vi "Write ADU Packet.vi"(8 "error in":errorcluster, 9 "modbus data unit":refnum<class "Modbus Data Unit.lvclass">, 10 "protocol layer":refnum<class "Network Protocol.lvclass">, 11 "transmission data unit in":refnum<class "Transmission Data Unit.lvclass">) -> (0 "error out":errorcluster, 2 "protocol layer out":refnum<class "Network Protocol.lvclass">, 3 "transmission data unit out":refnum<class "Transmission Data Unit.lvclass">)   [LabVIEW 2012, in "Transmission Data Unit.lvclass"]
doc: "This method accepts a modbus modbus data unit as input and writes the data of the PDU onto the selected network."
uses:
  Transmission Data Unit.lvclass
  Modbus Data Unit/Modbus Data Unit.lvclass
  Network Protocol/Network Protocol.lvclass
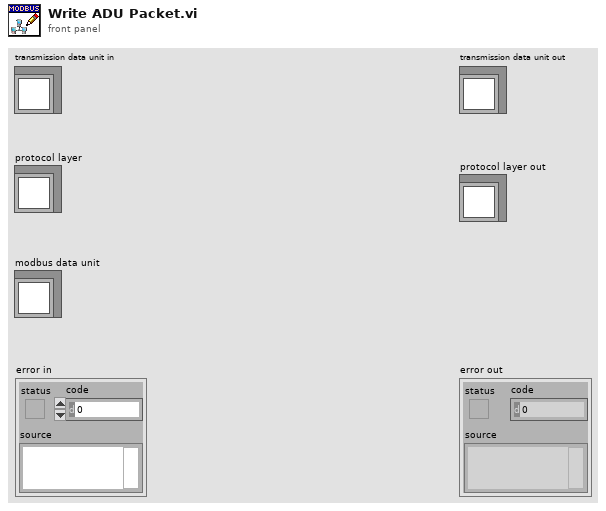
[diagram p1: front panel]
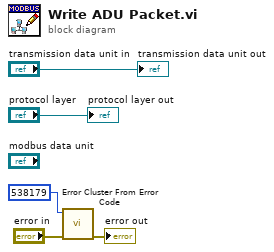
[diagram p0: block diagram]
diagram:
  n1 = call <vilib>:"Error Cluster From Error Code.vi"("error in (no error)"="error in", "error code (0)"=538179) -> ("error out"=→"error out":errorcluster)  [unwired: 7 in]
  "transmission data unit out" <- "transmission data unit in"
  "protocol layer out" <- "protocol layer"
